vi "Work.vi"(5 "Tag":T2, 6 "State in":T1, 7 "Init":T3, 10 "In":dbl, 11 "Action":T4) -> (0 "Error":errorcluster, 3 "Out":dbl, 4 "State out":T1)   [LabVIEW 2020, in "Worker Template.lvlib"]
uses:
  Worker Template.lvlib
  Block/FlexBlocks/Worker Action.ctl
  Init.ctl
  Tags.ctl
  State.ctl
  Block/FlexBlocks/FlexBlocks.lvlib
panel:
  # "To change the name that shows up when a worker is set in a FlexBlock, change the Window Title in the appearance settings of this VI's properties. Ctrl+i to access the properties or File Menu -> VI Properties."
  # "Other controls and indicators can be added to the connector pane as needed and will utilize lossless communication with other Workers and loops. Any inputs that do not require lossless inputs, such as configuration parameters that only care about latest values, should be added to the Tags input cluster and not directly connected to the connector pane.\n\nLocation does not matter for any control or indicator on the connector pane however the pre-defined elements on this template must keep their starting labels."
  # "The connector pane pattern can be changed if more terminals are needed for the worker."
  # "The Action input tells the worker whether it is the first run of the worker with \"Start\", is a \"Work\" iteration, or if execution is ending with \"Stop\".\n\nDuring Start and Stop calls, outputs are ignored. Start and Stop should rely solely on the values in Init and State in."
  # "Anything in a cluster named Init will be set once by FlexBlocks and remain static for all iterations."
  # "Setup the desired indicators for the FlexBlock to configure the output channels from the FlexBlock. This Out indicator can be replaced with the desired output type."
  # "Controls in a cluster named Tag will be broken out into separate FlexChannels and read with the latest value endpoint to be passed into the block."
  # "This In control is used to stream data into the worker each iteration and can be removed if there is no streamed input or changed to the desired data type."
  # "When an error is passed out of Error, the FlexBlock manager will stop running the worker. If the Manager UI is open, all blocks will be paused and the user has the option of attempting to continue or start single-stepping. If the Manager UI is not open then all workers will be stopped and execution will be ended."
  # "\"State in\" and \"State out\" are also special named clusters that the framework will maintain for the worker and pass the previous call's State out value as State in. During the Start action, State in will use default values, not the default values applied on the VI.\n\nUsage of State terminals is optional and if the VI is set to Preallocated Reentrancy, feedback nodes can be used instead. When used they must be named \"State in\" and \"State out\""
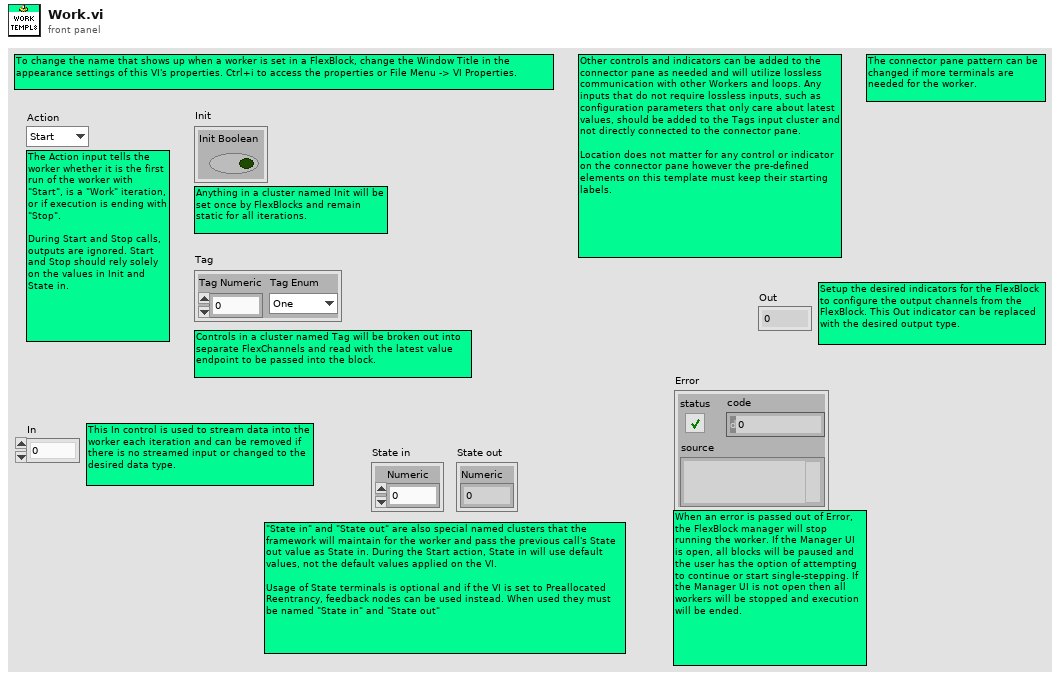
[diagram p1: front panel]
types:
  T1 = typedef "Worker Template.lvlib/State.ctl" = cluster{"Numeric":dbl}
  T2 = typedef "Worker Template.lvlib/Tags.ctl" = cluster{"Tag Numeric":dbl, "Tag Enum":enum16{"One", "Two", "Three"}}
  T3 = typedef "Worker Template.lvlib/Init.ctl" = cluster{"Init Boolean":bool}
  T4 = typedef "FlexBlocks.lvlib/Worker Action.ctl" = enum16{"Start", "Work", "Stop"}
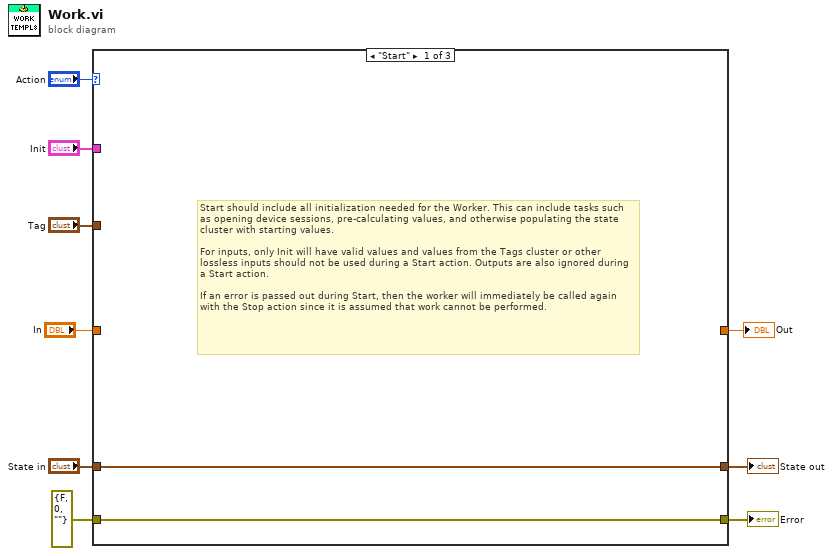
[diagram p0: block diagram]
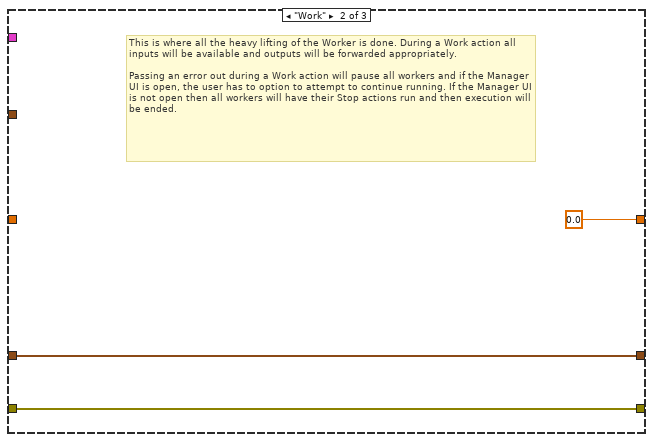
[diagram p2: hidden frame]
diagram:
  n1 = case shown="\"Start\"" "Action" {
    tunnel: "Init" -> [_ _ _]
    tunnel: "Tag" -> [_ _ _]
    tunnel: "State in" -> [w11 w14 w16]
    tunnel: [w11 w14 w16] -> w5
    tunnel: errorcluster {"status"=FALSE, "code"=0, "source"=""} ("error constant") -> [w10 w13 w15]
    tunnel: [w10 w13 w15] -> w3
    tunnel: "In" -> [_ _ _]
    tunnel: [_ 0.0 _] -> w1
    frame "Start" {
      # "Start should include all initialization needed for the Worker. This can include tasks such as opening device sessions, pre-calculating values, and otherwise populating the state cluster with starting values.\n\nFor inputs, only Init will have valid values and values from the Tags cluster or other lossless inputs should not be used during a Start action. Outputs are also ignored during a Start action.\n\nIf an error is passed out during Start, then the worker will immediately be called again with the Stop action since it is assumed that work cannot be performed."
    }
    frame "Work" {
      # "This is where all the heavy lifting of the Worker is done. During a Work action all inputs will be available and outputs will be forwarded appropriately.\n\nPassing an error out during a Work action will pause all workers and if the Manager UI is open, the user has to option to attempt to continue running. If the Manager UI is not open then all workers will have their Stop actions run and then execution will be ended."
    }
    frame "Stop" {
      # "The Stop action should be used to clean up any resources initialized in Start such as device sessions and other references.\n\nOutputs are ignored during a Stop action.\n\nIf an error is passed out during a Stop action, all other workers that may still be running will be paused and if the Manager UI is not displayed, execution will be ended. If the UI is open so the user can acknowledge the error they will also have the option to attempt to continue running the other workers."
    }
  }
  "State out" <- w5
  "Error" <- w3
  "Out" <- w1
